vi "crear memoria.vi"() -> ()   [LabVIEW 2020]
panel:
  out "IMAGEN BINARIZADA":picture
  out "MOMENTOS INVARIANTES DE HU":dbl[][](array[numeric])
  in  "NORMALIZACIÓN":bool=TRUE
  in  "INVERTIDO?":bool=TRUE
  in  "UMBRAL":u8(knob)=150 scale=0.0..255.0
  in  "CAPA DE COLOR":T1(ring)=enum."RGB2GRAY MATLAB"
  in  "Ruta":path
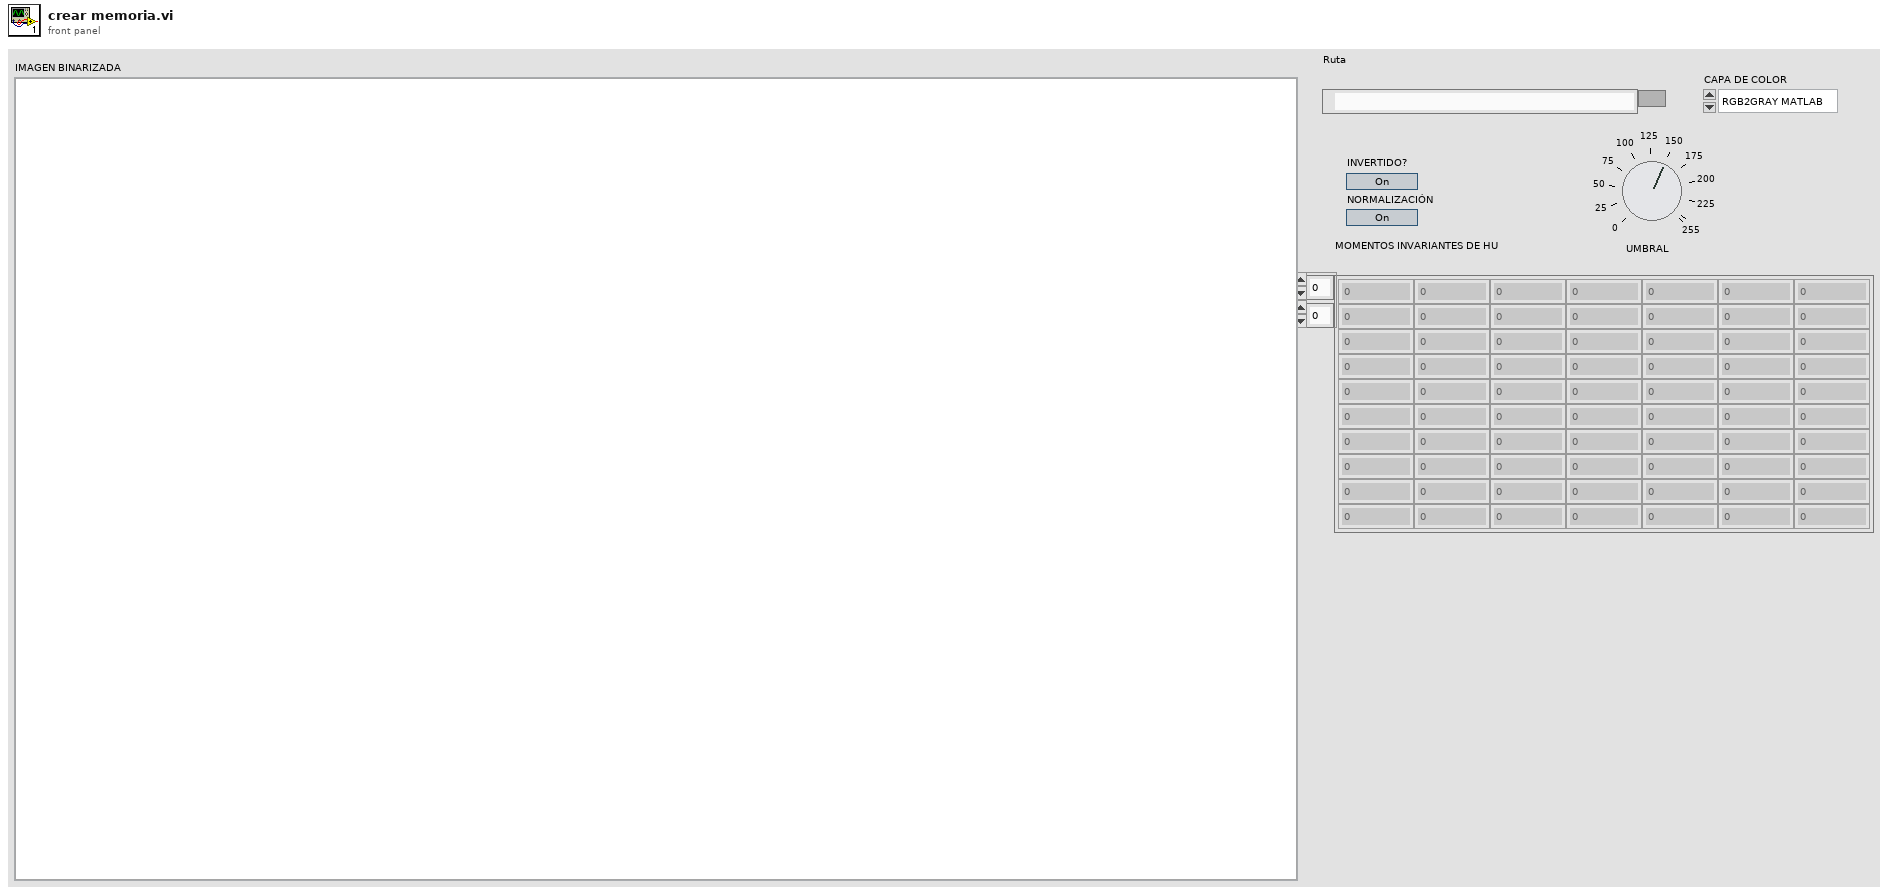
[diagram p1: front panel]
types:
  T1 = enum16{"H", "S", "V", "C", "M", "Y", "R", "G", "B", "RGB2GRAY MATLAB"}
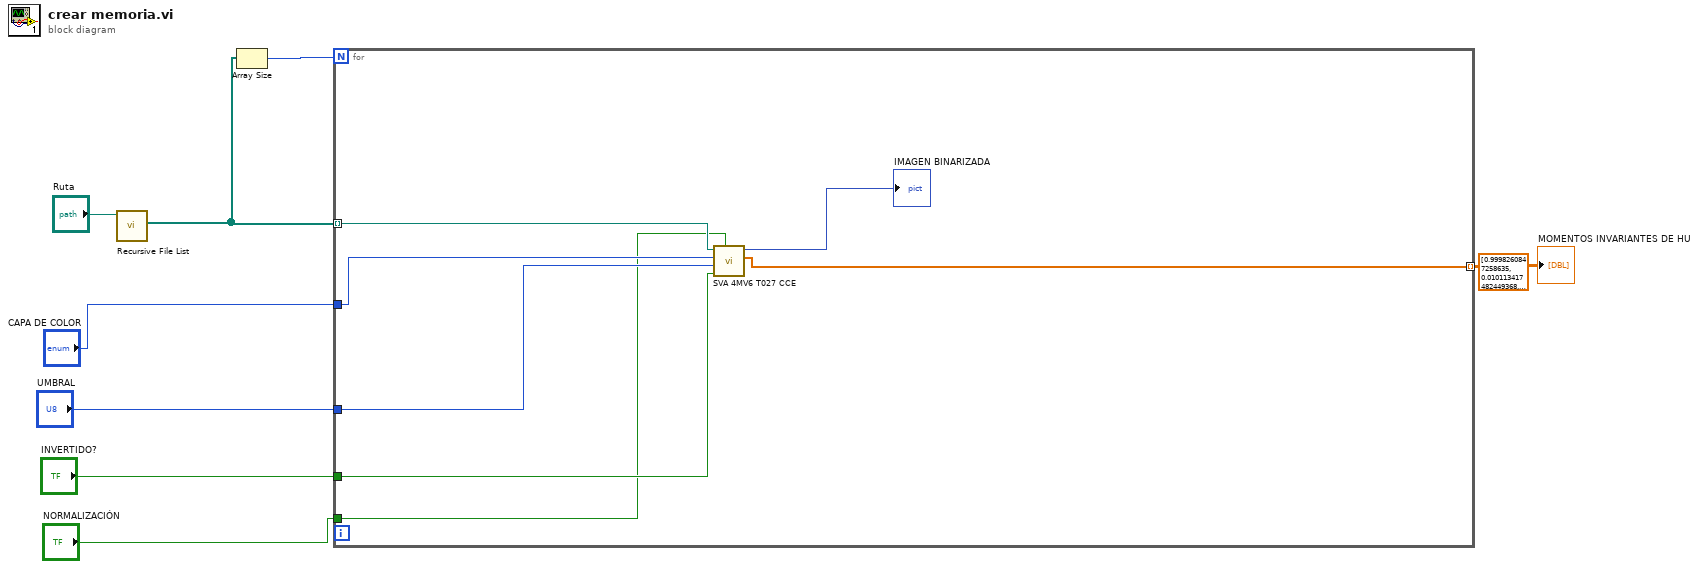
[diagram p0: block diagram]
diagram:
  (unwired) dbl[][] [[0.9998260847258635, 0.010113417482449368, 0.01557462856605164, 0.0017175592684488023, -4.872386513908903e-06, 4.374062218321611e-08, 1.5138885107619273e-07], [0.9872477986226894, 0.028071050355112787, 0.1004037020530345, 0.11992078296743537, 0.006302356185858303, 0.006795305469850189, 0.0024508780498351266], [0.9417468968058134, 0.310601353721232, 0.07481381332032479, 0.10432685636852428, 0.009212953693292327, 0.00806704104531403, 0.002902780203557166], [0.99293635887964, 0.11864790142642063, 0.00025024248305416993, 8.980454773548452e-06, 8.226357595102356e-11, -1.5362760148735018e-08, -8.194207686599058e-11], [0.9900416240435734, 0.13365702124311002, 0.044182211321199955, 0.001145617362205888, 4.3065833768968955e-06, 5.543788900167911e-05, 2.3031359982163546e-06], [0.9134316927738836, 0.4069919296519776, 6.798485878696647e-05, 0.000327432735967667, 2.7266678874394942e-08, 5.085841830259978e-07, -4.615581334935009e-10], [0.9240208783582403, 0.3823415571901731, 0.0005915014508827363, 1.137949687126939e-05, 3.957947747562796e-10, 2.1517264545494805e-08, 2.909795790518222e-10], [0.994765613853628, 0.09732221757456085, 0.03041456649378277, 0.006686772050812854, 2.6007594020255687e-05, 2.429188291092389e-06, -1.7390671348546814e-06], [0.9999997080867683, 0.0007640583488216332, 4.551103422565089e-06, 4.52827510295342e-06, -2.6965238360993628e-12, 4.7224332350655394e-09, 3.3275233672116626e-12], [0.9966873842602609, 0.08132807302127802, 4.16091732179383e-05, 2.9389523630263203e-05, 2.085257405688756e-10, -1.3144628336867574e-07, -9.814620585741512e-11]] ("MOMENTOS INVARIANTES DE HU")
  n1 = call <vilib>:"Recursive File List.vi"("Folder Path"="Ruta") -> ("All Files in Dir"=w8:path[])  [unwired: 6 in, 4 out]
  n2 = Array Size(array=w8) -> (size(s)=w7:i32)
  n3 = for {
    N: w7 -> [_]
    tunnel: w8 -> [w15] mode=indexing
    tunnel: "CAPA DE COLOR" -> [w12]
    tunnel: "UMBRAL" -> [w13]
    tunnel: "INVERTIDO?" -> [w14]
    tunnel: "NORMALIZACIÓN" -> [w11]
    tunnel: [w10] -> w1 mode=indexing
    n4 = call "SVA 4MV6 T027 CCE.vi"("NORMALIZACIÓN"=w11, "INVERTIDO?"=w14, "UMBRAL"=w13, "CAPA DE COLOR"=w12, "RUTA DE IMAGEN"=w15) -> ("MOMENTOS INVARIANTES DE HU"=w10:dbl[], "IMAGEN BINARIZADA"=→"IMAGEN BINARIZADA":picture)  [unwired: 5 in]
  }
  "MOMENTOS INVARIANTES DE HU" <- w1
